vi "_03_import a S-VI.vi"() -> ()   [LabVIEW 2020]
panel:
  in  "Enum":enum16{"Read Data", "Write Data"}(ring)
  out "error out":errorcluster
  in  "error in (no error)":errorcluster
  out "o/p":dbl
  in  "i/p":dbl
  # "Date : 17/03/25"
  # "Functional Global Variable (FGV)"
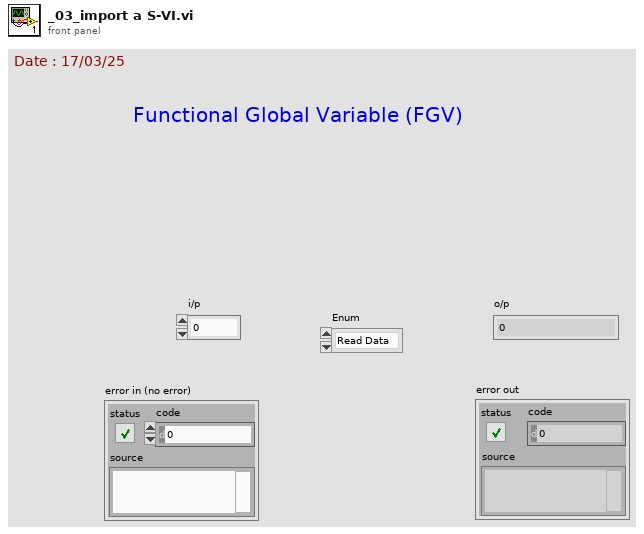
[diagram p1: front panel]
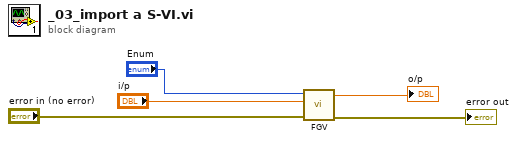
[diagram p0: block diagram]
diagram:
  n1 = call "FGV.vi"("Enum"="i/p", "error in (no error)"="error in (no error)", "i/p"="Enum") -> ("error out"=→"error out":errorcluster, "o/p"=→"o/p":dbl)  [unwired: 7 in]
